vi "Normalize.vi"(11 "Input":sgl[](array[numeric])) -> (3 "Normalized":sgl[](array[numeric]))   [LabVIEW 2012]
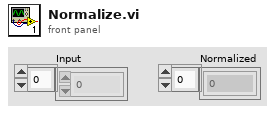
[diagram p1: front panel]
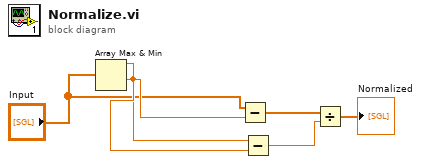
[diagram p0: block diagram]
diagram:
  n1 = Array Max & Min(array="Input") -> (max value=w3:sgl, min value=w4:sgl)  [unwired: 2 out]
  n2 = Subtract(x="Input", y=w4) -> (x-y=w2:sgl[])
  n3 = Subtract(x=w3, y=w4) -> (x-y=w5:sgl)
  n4 = Divide(x=w2, y=w5) -> (x/y=→"Normalized":sgl[])
